vi "RoundTripSpeedTest.vi"(8 "error in (no error)":errorcluster, 10 "Variant":variant, 11 "TestCase in":refnum<class "Python Data Tools Tests.lvclass">) -> (0 "error out":errorcluster, 1 "Elapsed Time (ms)":u32, 2 "Python String":string, 3 "TestCase out":refnum<class "Python Data Tools Tests.lvclass">, 4 "data":variant)   [LabVIEW 2020, in "Python Data Tools Tests.lvclass"]
uses:
  Python Data Tools Tests.lvclass
  source/jki_python_data_tools.lvlib
  <userlib>/_OpenG.lib/time/time.llb/openg_time.lvlib
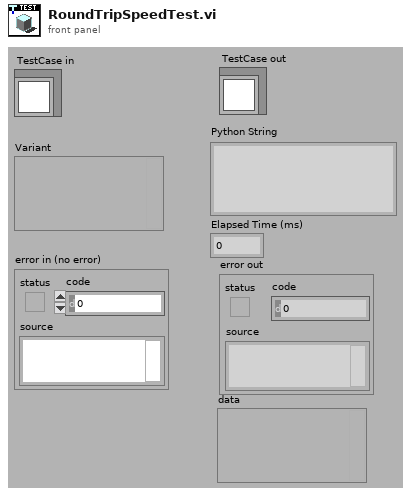
[diagram p1: front panel]
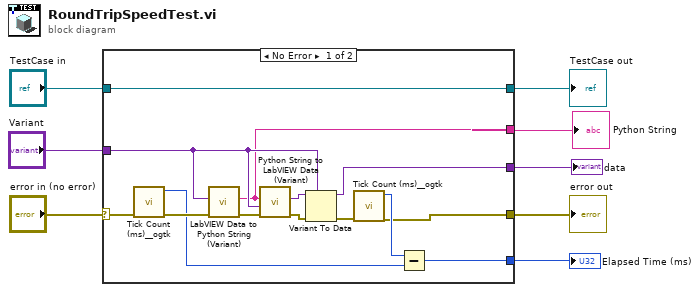
[diagram p0: block diagram]
diagram:
  n1 = case shown="No Error" "error in (no error)" {
    selector: "error in (no error)" -> [w17 w24]
    tunnel: "TestCase in" -> [w11 w23]
    tunnel: [w11 w23] -> w5
    tunnel: [w10 w24] -> w6
    tunnel: "Variant" -> [w19 _]
    tunnel: [w18 _] -> w3
    tunnel: [w12 _] -> w2
    tunnel: [w9 _] -> w1
    frame No Error {
      n2 = call <userlib>:"Tick Count (ms)__ogtk.vi"("error in (no error)"=w17) -> ("error out"=w16:errorcluster, "millisecond timer value"=w13:u32)  [unwired: 9 in]
      n3 = call "LabVIEW Data to Python String (Variant).vi"("error in (no error)"=w16, "LabVIEW Data"=w19) -> ("error out"=w22:errorcluster, "Python String"=w18:string)  [unwired: 8 in]
      n4 = call "Python String to LabVIEW Data (Variant).vi"("error in (no error)"=w22, "type"=w19, "Python String"=w18) -> ("error out"=w20:errorcluster, "LabVIEW Data"=w21:variant)  [unwired: 7 in]
      n5 = Variant To Data(error in=w20, type=w19, Variant=w21) -> (data=w9:variant, error out=w15:errorcluster)
      n6 = call <userlib>:"Tick Count (ms)__ogtk.vi"("error in (no error)"=w15) -> ("error out"=w10:errorcluster, "millisecond timer value"=w14:u32)  [unwired: 9 in]
      n7 = Subtract(x=w14, y=w13) -> (x-y=w12:u32)
    }
    frame Error {
    }
  }
  "error out" <- w6
  "TestCase out" <- w5
  "Python String" <- w3
  "Elapsed Time (ms)" <- w2
  "data" <- w1
